vi "Image Acquiring Module.vi"(7 "Scan Status in":T1, 8 "Error in":errorcluster) -> (0 "Error Out":errorcluster)   [LabVIEW 2018]
uses:
  Controls/scan status.ctl
  Controls/FGV Actions.ctl
  Controls/Save Bline to Mem Control.ctl
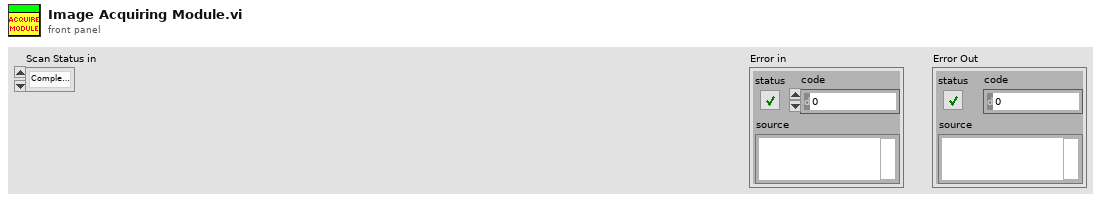
[diagram p1: front panel]
types:
  T1 = typedef "scan status.ctl" = enum16{"Complete Scan(ThorOCT)", "Complete Scan(PSOCT)", "Start(ThorOCT Spatial)", "Start(ThorOCT Spectral)", "Start(GPU FFT)", "Start(Alazar FFT)", "Scan(ThorOCT Spatial)", "Scan(ThorOCT Spectral)", "Scan(GPU FFT)", "Scan(Alazar FFT)", "Finish Scan(ThorOCT)", "Finish Scan(PSOCT)", "Scan(simulate)", "Start(ROI)", "Finish DO", "Scan DO", "Start DO"}
  T2 = typedef "FGV Actions.ctl" = enum16{"Init", "Set", "Get", "Clear"}
  T3 = typedef "System Parameters.ctl" = cluster{"Optical Parameters":T4, "Vibratome":T5, "Table Stages":T6, "Imaging Parameter":T9, "Galvo HW Parameters":cluster{"Analog Out Channel":tag, "Min Voltage":dbl, "Max Voltage":dbl, "Pixel Clock Source":tag, "Sample Rate":dbl, "Line Clock Out Ch":tag, "2P ready check":tag}, "Alazar parameters":T11, "Mosaic Paramter":T18, "Manual Controls":T19, "Z stage setting":T23, "Attenuator":T24, "Pause?":bool}
  T4 = typedef "Optical Parameters.ctl" = cluster{"Obj. Focal Length [mm]":dbl, "Scan Lens EFL[mm]":dbl, "Tube Lens EFL[mm]":dbl, "Galvo V Range (+/-)":dbl, "Galvo Max Half Angle [Deg]":dbl, "Max Galvo Range[%]":dbl}
  T5 = typedef "Vibratome Parameters.ctl" = cluster{"Pre Cut Dwell [s]":dbl, "Blade Frequency [RPM]":u16, "Slice Speed [mm/s]":dbl, "Post Cut Dwell [s]":dbl, "Ramp Time [s]":dbl, "Start X [mm]":dbl, "Start Y [mm]":dbl, "Slice Length [mm]":dbl, "Slice Axis":enum16{"X Axis", "Y Axis", "Z Axis"}, "Controller VISA Ref":refnum<visa-resource-name>}
  T6 = typedef "Translation Stage Parameters.ctl" = cluster{"X Stage":T7, "Y Stage":T7, "Z Stage":T7, "Attenuator":T7}
  T7 = typedef "Translation Stage Cluster.ctl" = cluster{"Position":dbl, "Is.Enabled?":bool, "Is.Connected?":bool, "Device SN":string, "AccelerationMaximum":dbl, "VelocityMaximum":dbl, "Acceleration":dbl, "Velocity":dbl, "waitTimeout (ms)":i32, "Model":T8, "Is.Homed?":bool, "MOVE":bool}
  T8 = typedef "Translation Stage Types.ctl" = enum16{"None", "Thorlabs LTS", "Thorlabs MLJ"}
  T9 = typedef "Imaging Parameters.ctl" = cluster{"Raster Scan Direction":T10, "Pixel Dwell Time [Clock Cycles]":u16, "Flyback Time [Clock Cycles]":u16, "XY Center [um]":cluster{"X":dbl, "Y":dbl}, "Pixel Step Size [um] X":dbl, "XY Image Size":enum16{"32 x 32", "64 x 64", "128 x 128", "256 x 256", "512 x 512", "1024 x 1024", "2048 x 2048"}, "Custom":bool, "Custom Size":cluster{"X":u16, "Y":u16}, "Line Averages":u16, "Pixel Step Size [um] Y":dbl}
  T10 = typedef "Scan Direction.ctl" = enum16{"Uni Directional", "Bi Directional", "None"}
  T11 = typedef "Alazar parameters.ctl" = cluster{"Trigger Settings":cluster{"General Trigger Settings":T12, "Trigger Engine 1":T13, "Trigger Engine 2":T13}, "Device ID":T14, "Ch A Input Control":T15, "Ch B Input Control":T15, "Acq Settings":T16, "Capture Clock":T17}
  T12 = typedef "General Trigger Settings.ctl" = cluster{"Trigger Operation":u32, "Coupling ID":u32, "Range ID":u32, "Delay":u32, "Timeout Ticks":u32, "Mode":u32, "Parameter":u32}
  T13 = typedef "Trigger Engine Controls.ctl" = cluster{"Trigger Engine":u32, "Source":u32, "Slope":u32, "Level":u32}
  T14 = typedef "Alazar Device ID.ctl" = cluster{"System ID":u32, "Board ID":u32}
  T15 = typedef "Channel Input Controls.ctl" = cluster{"Channel":u8, "Coupling":u32, "Range":u32, "Impedance":u32}
  T16 = typedef "Alazar Acquisition Settings.ctl" = cluster{"Record Length":u32, "Offset":u32, "Records Per Buffer":u32, "Records Count (Records/Acq)":u32, "Window Type":u32, "Footer":u32, "Samples per record":u32, "Output Format":u32}
  T17 = typedef "Clock Controls.ctl" = cluster{"Sample Rate":u32, "Decimation":u32, "Source":u32, "Edge":u32}
  T18 = typedef "Mosaic Parameter.ctl" = cluster{"X Axis":cluster{"Start [mm]":dbl, "Steps [pts]":dbl, "End [mm]":dbl}, "Y Axis":cluster{"Start [mm]":dbl, "Steps [pts]":dbl, "End [mm]":dbl}, "Scan Pattern":enum16{"Uni-directional", "Bi-Directional", "Spiral Out", "Spiral In"}, "Overlap Options":cluster{"Overlap Type":enum16{"No Overlap", "X Only", "Y Only", "X and Y"}, "Percent Overlap":u8, "Justify":enum16{"Start", "Center", "End"}}}
  T19 = typedef "Manual Controls.ctl" = cluster{"Data Path":path, "Save parameters":T20, "Acquisition mode":T21, "PSOCT Channel":u32, "Save data?":bool, "AIP rotation angle":dbl, "Outgoing Mail Server (SMTP)":string, "Email":string, "Password":string, "Carrier 1":enum16{"T-Mobile", "AT&T", "Verizon", "Sprint"}, "phone number 1":string, "Subject":string, "Message":string, "Carrier 2":enum16{"T-Mobile", "AT&T", "Verizon", "Sprint"}, "phone number 2":string, "Outputs for GPU FFT":T22, "First Slice #":i32}
  T20 = typedef "FFT parameters.ctl" = cluster{"start pixel":i32, "#pixels to save":i32}
  T21 = typedef "FFT mode.ctl" = enum16{"ThorOCT B line", "ThorOCT Spectral", "ThorOCT FFT", "Alazar B line", "Alazar FFT", "GPU FFT", "Alazar Spectral", "Simulation", "auto adjust focus", "Save all"}
  T22 = typedef "GPU FFT outputs.ctl" = enum16{"Amp + Phase diff", "Amp + Phase", "Amp only"}
  T23 = typedef "Vibratome Param.ctl" = cluster{"first cut height(mm)":dbl, "cut thickness[um]":u32[], "#cycles":u16, "PSOCT thickness(um)":u32[], "First image height(mm)":dbl, "Pause?":bool[], "Z0":dbl, "fixed Z0?":bool, "Cut_aft_2P?(leave empty if no 2P)":bool[], "2P thickness(um) (leave empty if not used)":u32[], "2P_cover_all_depth? (leave empty if no 2P)":bool[]}
  T24 = typedef "attenuator.ctl" = cluster{"Power after Objective (recalibrate every 6 month)":dbl[]}
  T25 = typedef "Save Bline to Mem Control.ctl" = enum16{"Output data", "Save(ThorOCT)", "Save(PSOCT)", "FFT and Save", "Uninit", "PSOCT Spectral buffer Set", "PSOCT Spatial buffer Set", "PSOCT Spectral buffer Init", "PSOCT Spatial buffer Init", "ThorOCT Spectral buffer Init", "ThorOCT Spatial buffer Init", "ThorOCT Spectral buffer Set", "ThorOCT Spatial buffer Set", "ThorOCT Spectral Save", "Alazar Spectral Save", "PSOCT save all", "Average"}
  T26 = typedef "ScanType.ctl" = enum16{"Single Frame", "Continuous Frame", "ROI Line", "Vibratome", "Mosaic", "Mosaic + Slice"}
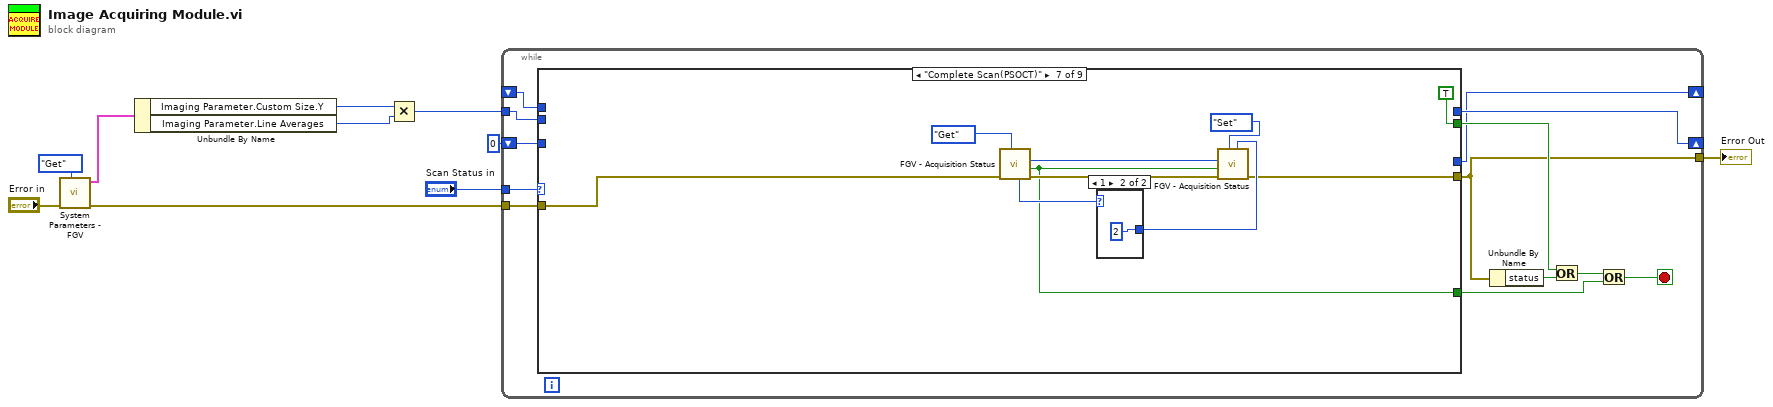
[diagram p0: block diagram]
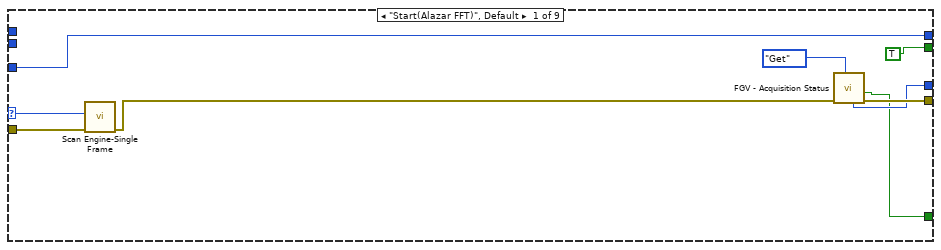
[diagram p2: hidden frame]
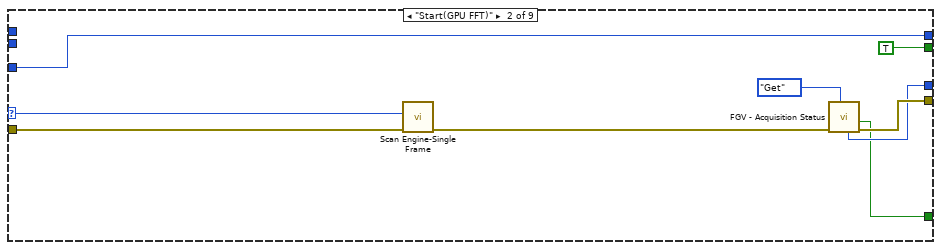
[diagram p3: hidden frame]
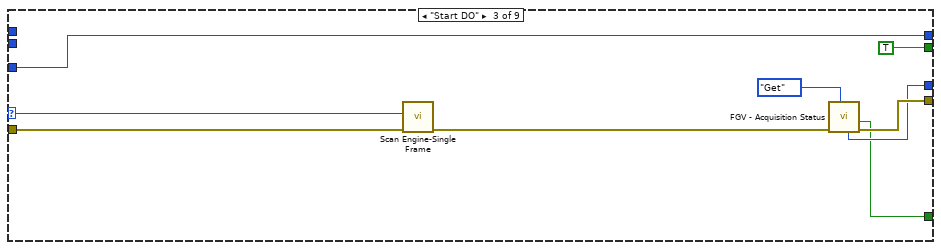
[diagram p4: hidden frame]
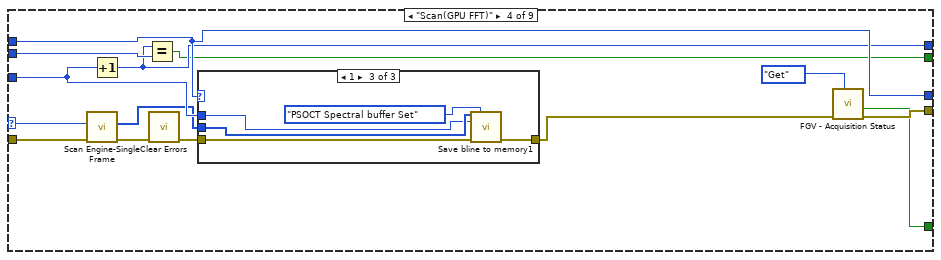
[diagram p5: hidden frame]
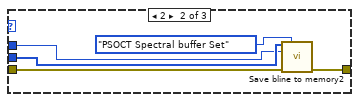
[diagram p7: hidden frame]
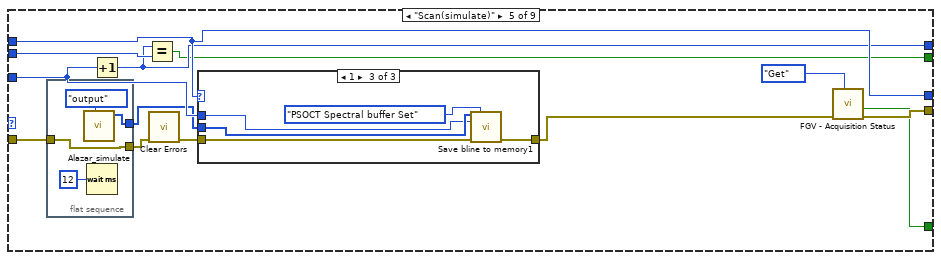
[diagram p8: hidden frame]
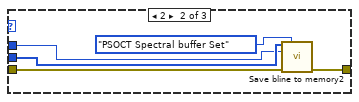
[diagram p10: hidden frame]
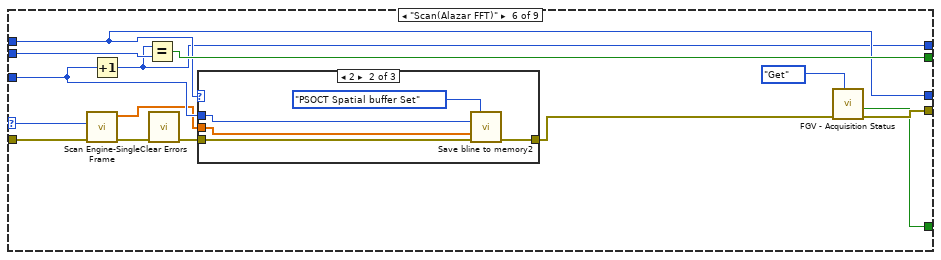
[diagram p11: hidden frame]
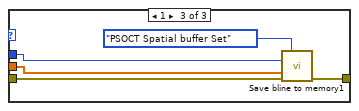
[diagram p13: hidden frame]
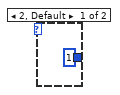
[diagram p14: hidden frame]
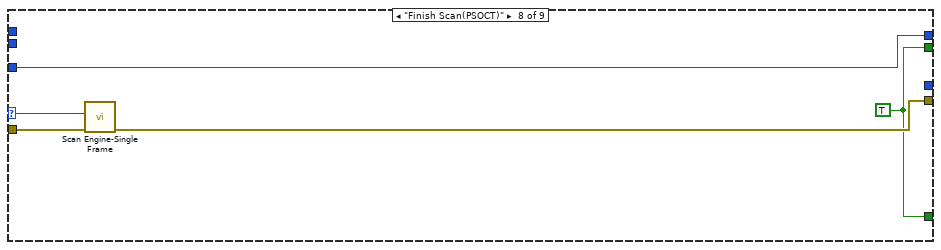
[diagram p15: hidden frame]
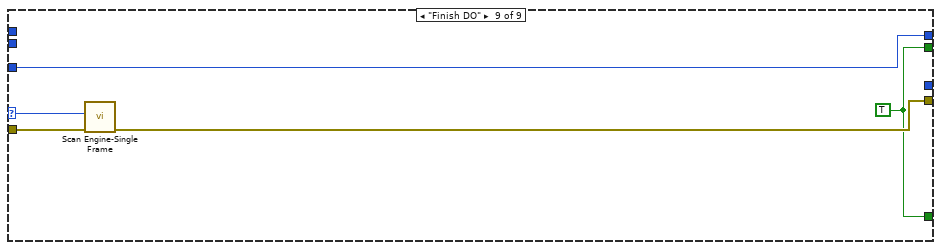
[diagram p16: hidden frame]
diagram:
  n1 = call "System Parameters - FGV.vi"("Actions"=FGV_Actions."Get", "Error In"="Error in") -> ("Error Out"=w2:errorcluster, "System Parameters [Out]"=w3:T3)  [unwired: 8 in]
  n2 = Unbundle By Name(w3) -> ("Imaging Parameter.Custom Size.Y"=w7:u16, "Imaging Parameter.Line Averages"=w6:u16)
  n3 = Multiply(x=w7, y=w6) -> (x*y=w5:u16)
  n4 = while {
    tunnel: w2 -> [w21]
    tunnel: "Scan Status in" -> [w23]
    shift-right: [w22] -> _
    shift-left: u32 0 ("bline count") -> [w19]
    tunnel: w5 -> [w16]
    shift-right: [w14] -> _
    shift-left: _ -> [w15]
    tunnel: [w13] -> w8
    stop <- w17 stop-if-true
    n5 = case shown="\"Complete Scan(PSOCT)\"" w23 {
      selector: w23 -> [w29 w39 w48 w58 _ w116 _ w142 w147]
      tunnel: w21 -> [w32 w41 w50 w59 w77 w117 w136 w145 w150]
      tunnel: [w26 w35 w44 w54 w81 w108 w129 w143 w148] -> w13
      tunnel: [TRUE TRUE TRUE w60 w84 w113 TRUE ("task done?") w141 w146] -> w20
      tunnel: w19 -> [w30 w40 w49 w61 w85 w115 _ w144 w149]
      tunnel: [w30 w40 w49 w62 w86 w111 _ w144 w149] -> w22
      tunnel: w16 -> [_ _ _ w63 w87 w114 _ _ _]
      tunnel: w15 -> [_ _ _ w64 w88 w112 _ _ _]
      tunnel: [w25 w34 w43 w64 w88 w112 _ _ _] -> w14
      tunnel: [w24 w33 w42 w53 w80 w107 w131 w141 w146] -> w11
      frame "Start(Alazar FFT)", Default {
        n6 = call "Scan Engine-Single Frame.vi"("Error in"=w32, "Scan Status in"=w29) -> ("Error Out"=w27:errorcluster)  [unwired: 7 in, 2 out]
        n7 = call "FGV - Acquisition Status.vi"("Actions"=FGV_Actions."Get", "Error In"=w27) -> ("Error Out"=w26:errorcluster, "Quit status out"=w24:bool, "mem loc out"=w25:i32)  [unwired: 6 in, 1 out]
      }
      frame "Start(GPU FFT)" {
        n8 = call "Scan Engine-Single Frame.vi"("Error in"=w41, "Scan Status in"=w39) -> ("Error Out"=w36:errorcluster)  [unwired: 7 in, 2 out]
        n9 = call "FGV - Acquisition Status.vi"("Actions"=FGV_Actions."Get", "Error In"=w36) -> ("Error Out"=w35:errorcluster, "Quit status out"=w33:bool, "mem loc out"=w34:i32)  [unwired: 6 in, 1 out]
      }
      frame "Start DO" {
        n10 = call "Scan Engine-Single Frame.vi"("Error in"=w50, "Scan Status in"=w48) -> ("Error Out"=w45:errorcluster)  [unwired: 7 in, 2 out]
        n11 = call "FGV - Acquisition Status.vi"("Actions"=FGV_Actions."Get", "Error In"=w45) -> ("Error Out"=w44:errorcluster, "Quit status out"=w42:bool, "mem loc out"=w43:i32)  [unwired: 6 in, 1 out]
      }
      frame "Scan(GPU FFT)" {
        n12 = call "Scan Engine-Single Frame.vi"("Error in"=w59, "Scan Status in"=w58) -> ("Error Out"=w52:errorcluster, "Buffer"=w57:u16[])  [unwired: 7 in, 1 out]
        n13 = Increment(x=w61) -> (x+1=w62:u32)
        n14 = Equal?(x=w62, y=w63) -> (x = y?=w60:bool)
        n15 = call <vilib>:"Clear Errors.vi"("error in (no error)"=w52) -> ("error out"=w51:errorcluster)  [unwired: 5 in, 1 out]
        n16 = case shown="1" w64 {
          tunnel: w51 -> [w65 w70 w75]
          tunnel: [w65 w69 w74] -> w55
          tunnel: w61 -> [_ w66 w72]
          tunnel: w57 -> [_ w67 w73]
          frame 0, Default {
          }
          frame 2 {
            n17 = call "Save bline to memory2.vi"("PSOCTSpectral Bline"=w67, "action"=Save_Bline_to_Mem_Control."PSOCT Spectral buffer Set", "index (row)"=w66, "error in"=w70) -> ("error out"=w69:errorcluster)  [unwired: 11 in]
          }
          frame 1 {
            n18 = call "Save bline to memory1.vi"("PSOCTSpectral Bline"=w73, "action"=Save_Bline_to_Mem_Control."PSOCT Spectral buffer Set", "index (row)"=w72, "error in"=w75) -> ("error out"=w74:errorcluster)  [unwired: 11 in]
          }
        }
        n19 = call "FGV - Acquisition Status.vi"("Actions"=FGV_Actions."Get", "Error In"=w55) -> ("Error Out"=w54:errorcluster, "Quit status out"=w53:bool)  [unwired: 6 in, 2 out]
      }
      frame "Scan(simulate)" {
        n20 = flat-sequence {
          tunnel: [w92] -> w78
          tunnel: w77 -> [w90]
          tunnel: [w90] -> w76
          frame #0 {
            n21 = call "Alazar_simulate.vi"("Enum"=enum16{"init", "output"}."output") -> ("Array"=w92:u16[])  [unwired: 10 in]
            n22 = Wait (ms)(milliseconds to wait=u32 12) -> ()  [unwired: 1 out]
          }
        }
        n23 = Increment(x=w85) -> (x+1=w86:u32)
        n24 = Equal?(x=w86, y=w87) -> (x = y?=w84:bool)
        n25 = call <vilib>:"Clear Errors.vi"("error in (no error)"=w76) -> ("error out"=w79:errorcluster)  [unwired: 5 in, 1 out]
        n26 = case shown="1" w88 {
          tunnel: w79 -> [w93 w98 w103]
          tunnel: [w93 w97 w102] -> w82
          tunnel: w85 -> [_ w94 w100]
          tunnel: w78 -> [_ w95 w101]
          frame 0, Default {
          }
          frame 2 {
            n27 = call "Save bline to memory2.vi"("PSOCTSpectral Bline"=w95, "action"=Save_Bline_to_Mem_Control."PSOCT Spectral buffer Set", "index (row)"=w94, "error in"=w98) -> ("error out"=w97:errorcluster)  [unwired: 11 in]
          }
          frame 1 {
            n28 = call "Save bline to memory1.vi"("PSOCTSpectral Bline"=w101, "action"=Save_Bline_to_Mem_Control."PSOCT Spectral buffer Set", "index (row)"=w100, "error in"=w103) -> ("error out"=w102:errorcluster)  [unwired: 11 in]
          }
        }
        n29 = call "FGV - Acquisition Status.vi"("Actions"=FGV_Actions."Get", "Error In"=w82) -> ("Error Out"=w81:errorcluster, "Quit status out"=w80:bool)  [unwired: 6 in, 2 out]
      }
      frame "Scan(Alazar FFT)" {
        n30 = call "Scan Engine-Single Frame.vi"("Error in"=w117, "Scan Status in"=w116) -> ("Error Out"=w105:errorcluster, "FFT Buffer"=w104:sgl[])  [unwired: 7 in, 1 out]
        n31 = Increment(x=w115) -> (x+1=w111:u32)
        n32 = Equal?(x=w111, y=w114) -> (x = y?=w113:bool)
        n33 = call <vilib>:"Clear Errors.vi"("error in (no error)"=w105) -> ("error out"=w106:errorcluster)  [unwired: 5 in, 1 out]
        n34 = case shown="2" w112 {
          tunnel: w106 -> [w118 w120 w125]
          tunnel: [w118 w119 w124] -> w109
          tunnel: w115 -> [_ w123 w127]
          tunnel: w104 -> [_ w122 w128]
          frame 0, Default {
          }
          frame 2 {
            n35 = call "Save bline to memory2.vi"("action"=Save_Bline_to_Mem_Control."PSOCT Spatial buffer Set", "index (row)"=w123, "PSOCT Spatial Bline"=w122, "error in"=w120) -> ("error out"=w119:errorcluster)  [unwired: 11 in]
          }
          frame 1 {
            n36 = call "Save bline to memory1.vi"("action"=Save_Bline_to_Mem_Control."PSOCT Spatial buffer Set", "index (row)"=w127, "PSOCT Spatial Bline"=w128, "error in"=w125) -> ("error out"=w124:errorcluster)  [unwired: 11 in]
          }
        }
        n37 = call "FGV - Acquisition Status.vi"("Actions"=FGV_Actions."Get", "Error In"=w109) -> ("Error Out"=w108:errorcluster, "Quit status out"=w107:bool)  [unwired: 6 in, 2 out]
      }
      frame "Complete Scan(PSOCT)" {
        n38 = call "FGV - Acquisition Status.vi"("Actions"=FGV_Actions."Get", "Error In"=w136) -> ("Error Out"=w133:errorcluster, "Quit status out"=w131:bool, "Scan Type [Out]"=w130:T26, "mem loc out"=w135:i32)  [unwired: 6 in]
        n39 = case shown="1" w135 {
          tunnel: [1 2] -> w132
          frame 2, Default {
          }
          frame 1 {
          }
        }
        n40 = call "FGV - Acquisition Status.vi"("mem loc"=w132, "Actions"=FGV_Actions."Set", "Error In"=w133, "Quit status"=w131, "Scan Type [In]"=w130) -> ("Error Out"=w129:errorcluster)  [unwired: 3 in, 3 out]
      }
      frame "Finish Scan(PSOCT)" {
        w141 = TRUE ("task done?")
        n41 = call "Scan Engine-Single Frame.vi"("Error in"=w145, "Scan Status in"=w142) -> ("Error Out"=w143:errorcluster)  [unwired: 7 in, 2 out]
      }
      frame "Finish DO" {
        w146 = TRUE ("task done?")
        n42 = call "Scan Engine-Single Frame.vi"("Error in"=w150, "Scan Status in"=w147) -> ("Error Out"=w148:errorcluster)  [unwired: 7 in, 2 out]
      }
    }
    n43 = Unbundle By Name(w13) -> ("status"=w12:bool)
    n44 = Or(x=w20, y=w12) -> (x .or. y?=w18:bool)
    n45 = Or(x=w18, y=w11) -> (x .or. y?=w17:bool)
  }
  "Error Out" <- w8
